vi "Event_log_example.vi"() -> ()   [LabVIEW 2017, in "labview-standard-library.lvlib"]
uses:
  labview-standard-library.lvlib
  Time&Event_cluster.ctl
  Event_type_selecter.ctl
panel:
  in  "Write txt/csv":bool
  out "element":T1
  in  "Warning":bool
  in  "Event":bool
  out "error out":errorcluster
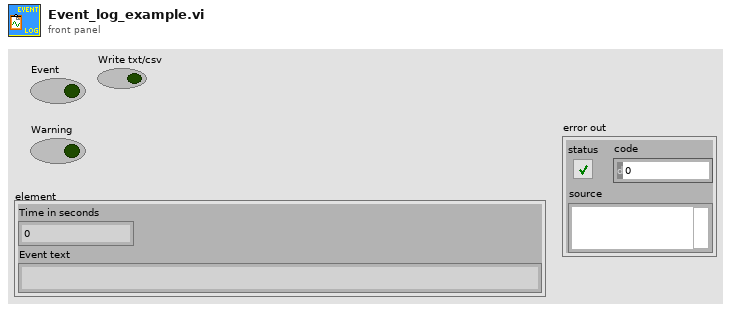
[diagram p1: front panel]
types:
  T1 = typedef "labview-standard-library.lvlib/Time&Event_cluster.ctl" = cluster{"Time in seconds":dbl, "Event text":string}
  T2 = typedef "labview-standard-library.lvlib/Event_type_selecter.ctl" = enum16{"Event", "Warning", "Write events"}
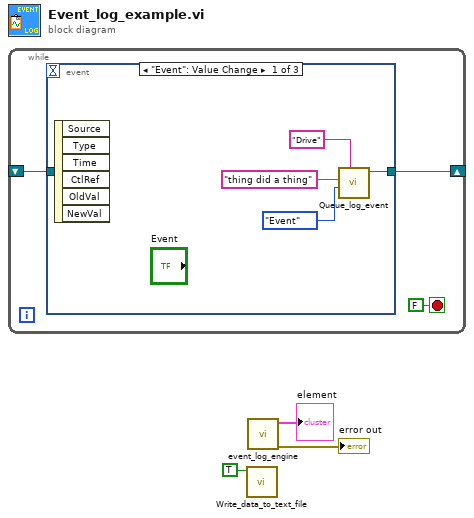
[diagram p0: block diagram]
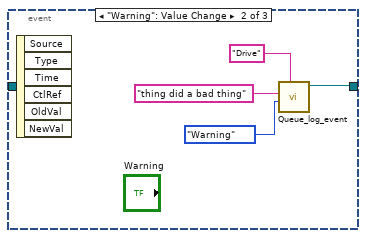
[diagram p2: hidden frame]
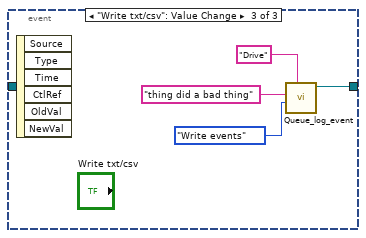
[diagram p3: hidden frame]
diagram:
  n1 = while {
    shift-right: [w6] -> _
    shift-left: _ -> [w5]
    stop <- FALSE stop-if-true
    n2 = event shown="[0] \"Event\": Value Change" {
      selector: _ -> [_ _ _]
      dyn-events: _ -> [_ _ _]
      timeout: _ -> [_ _ _]
      tunnel: w5 -> [_ _ _]
      tunnel: [w7 w11 w15] -> w6
      event "Event": Value Change {
        n3 = event-data() -> ()  [unwired: 1 in, 6 out]
        n4 = call "Queue_log_event.vi"("Subsystem name in"="Drive", "Event or Warning"=Event_type_selecter."Event", "Event discription in"="thing did a thing") -> ("queue out"=w7:refnum<queue>)  [unwired: 8 in]
      }
      event "Warning": Value Change {
        n5 = event-data() -> ()  [unwired: 1 in, 6 out]
        n6 = call "Queue_log_event.vi"("Subsystem name in"="Drive", "Event or Warning"=Event_type_selecter."Warning", "Event discription in"="thing did a bad thing") -> ("queue out"=w11:refnum<queue>)  [unwired: 8 in]
      }
      event "Write txt/csv": Value Change {
        n7 = event-data() -> ()  [unwired: 1 in, 6 out]
        n8 = call "Queue_log_event.vi"("Subsystem name in"="Drive", "Event or Warning"=Event_type_selecter."Write events", "Event discription in"="thing did a bad thing") -> ("queue out"=w15:refnum<queue>)  [unwired: 8 in]
      }
    }
  }
  n9 = call "Write_data_to_text_file.vi"(".CSV? (F=.txt)"=TRUE) -> ()  [unwired: 11 in]
  n10 = call "event_log_engine.vi"() -> ("error out"=→"error out":errorcluster, "element"=→"element":T1)  [unwired: 10 in]
